vi "CameraState.vi"(0 "Strings in":string[](array[string]), 1 "Dubs in":dbl[](array[numeric])) -> ()   [LabVIEW 2018]
panel:
  in  "subvi":bool=TRUE
  in  "CamState":dbl
  in  "CamFile":path=path "C:/CuspControl/GPIB and Network/Cusp/CameraState.txt"
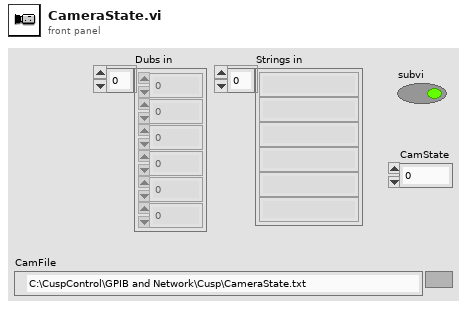
[diagram p1: front panel]
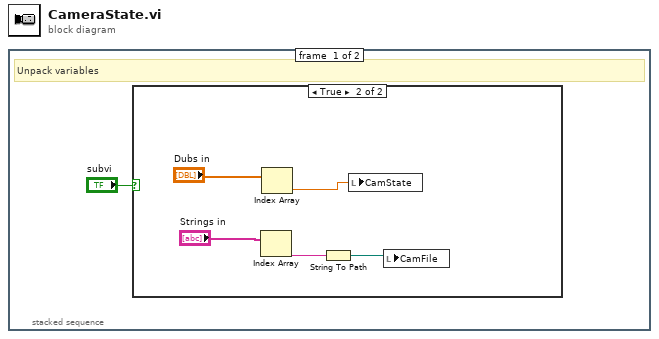
[diagram p0: block diagram]
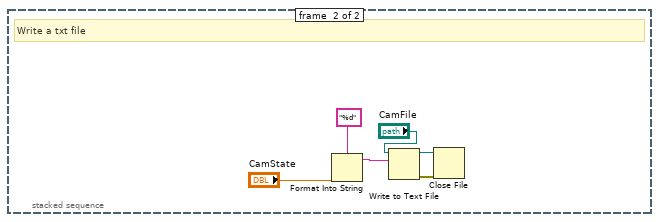
[diagram p3: hidden frame]
diagram:
  n1 = stacked-sequence {
    frame #0 {
      # "Unpack variables"
      n2 = case shown="True" "subvi" {
        frame False {
        }
        frame True {
          n3 = Index Array(array="Strings in") -> (element=w3:string)  [unwired: 1 in]
          n4 = Index Array(array="Dubs in") -> (element=w4:dbl)  [unwired: 1 in]
          n5 = String To Path(string=w3) -> (path=w2:path)
          n6 = local write "CamState"(w4) -> ()
          n7 = local write "CamFile"(w2) -> ()
        }
      }
    }
    frame #1 {
      # "Write a txt file"
      n8 = Format Into String(format string="%d", "CamState") -> (resulting string=w11:string)  [unwired: 2 in, 1 out]
      n9 = Write to Text File(file (use dialog)="CamFile", text=w11) -> (refnum out=w7:refnum<file>, error out=w8:errorcluster)  [unwired: 2 in, 1 out]
      n10 = Close File(refnum=w7, error in=w8) -> ()  [unwired: 2 out]
    }
  }
